vi "Create BF Steps 20220125.vi"(9 "Step_v":dbl=1.0, 10 "Stop_v":dbl=12.0 format="%#_13g", 11 "Start_v":dbl=10.0 format="%#_13g") -> (1 "BF Names":string[](array[string]), 2 "BF values":dbl[](array[numeric]), 3 "BFSamples":i32)   [LabVIEW 2013]
uses:
  <vilib>/Analysis/1siggen.llb/Ramp Pattern by Delta.vi
  <vilib>/Analysis/NI_AALBase.lvlib
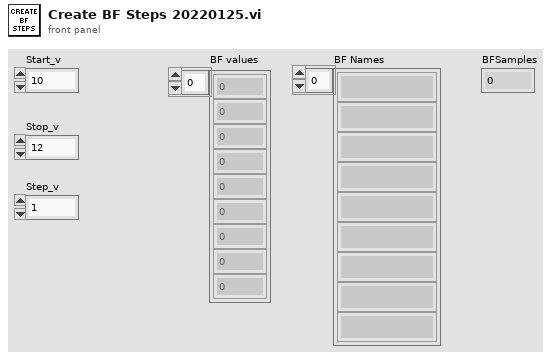
[diagram p1: front panel]
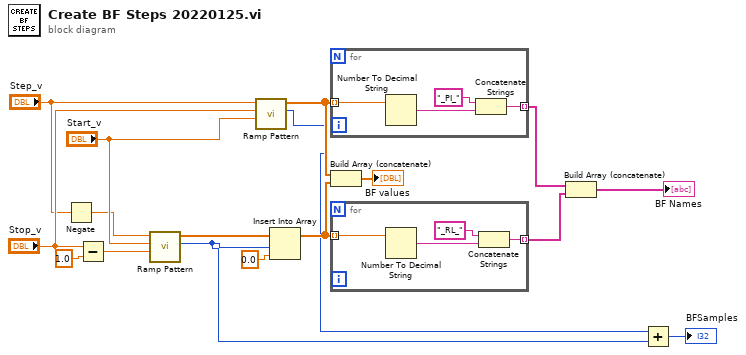
[diagram p0: block diagram]
diagram:
  n1 = Negate(x="Step_v") -> (-x=w12:dbl)
  n2 = Subtract(x="Stop_v", y=1.0) -> (x-y=w14:dbl)
  n3 = call-poly <vilib>:"Ramp Pattern.vi"("start"=w14, "end"="Start_v", "delta"=w12) -> ("samples"=w2:i32, "Ramp Pattern"=w9:dbl[])  [unwired: 6 in, 1 out]
  n4 = call-poly <vilib>:"Ramp Pattern.vi"("start"="Start_v", "end"="Stop_v", "delta"="Step_v") -> ("samples"=w3:i32, "Ramp Pattern"=w11:dbl[])  [unwired: 6 in, 1 out]
  n5 = Insert Into Array(array=w9, index=w2, new element=0.0 ("new element/subarray")) -> (w8:dbl[])
  n6 = for {
    tunnel: w11 -> [w21] mode=indexing
    tunnel: [w18] -> w6 mode=indexing
    n7 = Number To Decimal String(number=w21) -> (decimal integer string=w19:string)  [unwired: 1 in]
    n8 = Concatenate Strings("_PI_" ("string"), w19) -> (w18:string)
  }
  n9 = Build Array (concatenate)(w11, w8) -> (→"BF values":dbl[])
  n10 = for {
    tunnel: w8 -> [w25] mode=indexing
    tunnel: [w22] -> w5 mode=indexing
    n11 = Number To Decimal String(number=w25) -> (decimal integer string=w23:string)  [unwired: 1 in]
    n12 = Concatenate Strings("_RL_" ("string"), w23) -> (w22:string)
  }
  n13 = Build Array (concatenate)(w6, w5) -> (→"BF Names":string[])
  n14 = Add(x=w3, y=w2) -> (x+y=→"BFSamples":i32)
